vi "Open TDMS.vi"(11 "RevPath":path=path "E:/Data" caption="TDMS Path") -> (0 "TDMS File Found":bool, 2 "RevPath out":path=path "E:/Data" caption="TDMS Path", 3 "tdms file out":refnum<k34>)   [LabVIEW 2020]
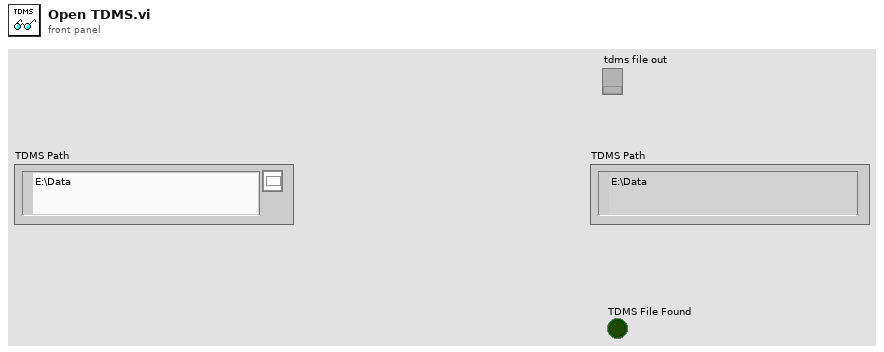
[diagram p1: front panel]
types:
  T1 = enum16{"open", "open or create", "create or replace", "create", "open (read-only)"}
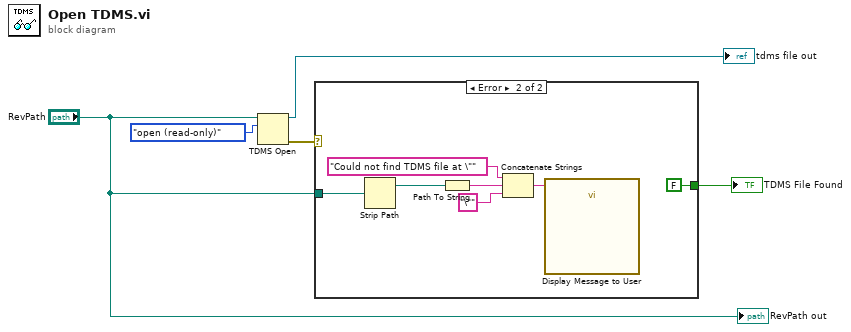
[diagram p0: block diagram]
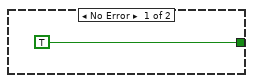
[diagram p2: hidden frame]
diagram:
  n1 = TDMS Open(10:T1."open (read-only)" ("operation (0:open)"), 11:"RevPath") -> (0:w3:errorcluster, 3:→"tdms file out":refnum<k34>)  [unwired: 5 in]
  n2 = case shown="Error" w3 {
    tunnel: [TRUE ("OK") FALSE ("OK")] -> w4
    tunnel: "RevPath" -> [_ w10]
    frame No Error {
    }
    frame Error {
      n3 = Strip Path(path=w10) -> (stripped path=w9:path)  [unwired: 1 out]
      n4 = Path To String(path=w9) -> (string=w13:string)
      n5 = Concatenate Strings("Could not find TDMS file at \"" ("string"), w13, "\"" ("string")) -> (w11:string)
      n6 = call "Display Message to User"("Message"=w11) -> ()  [unwired: 9 in, 2 out]
    }
  }
  "TDMS File Found" <- w4
  "RevPath out" <- "RevPath"
